vi "UHR-Fleezers Control (fpga) - 10.7.vi"() -> ()   [LabVIEW 2014]
doc: "UHR-Fleezers Instrument Control Code (fpga)"
uses:
  <vilib>/eio/EIONode/EIONode.xnode
  <vilib>/eio/EIOMethodNode/EIOMethodNode.xnode
  <vilib>/rvi/DataTransferAndStorage/Container/XNode/niFpgaContainer.xnode
  <vilib>/Platform/TimedLoop/XDataNode/XDataNode.xnode
  <vilib>/Platform/TimedLoop/XDataNode/nitl_modes.ctl
  <vilib>/Platform/TimedLoop/XDataNode/XDNodeRunTimeDep.lvlib
  <vilib>/Platform/TimedLoop/XDataNode/wakeup.ctl
  <vilib>/Platform/TimedLoop/XDataNode/timing_clust.ctl
  <vilib>/addons/control/pid/fpga.llb/XNode/niFpgaPID.xnode
  <vilib>/rvi/eio/common/nirviEmuTemplateMethod_errors.vi
  <vilib>/rvi/interface/RandomDataEmulation/nirviRandomDataFpgaReadWriteTemplate.vi
panel:
  in  "Connector0/AO6":i16
  in  "Tab Control":T1(tab)=enum."Force FB"
  in  "Trap Pos to FIFO":bool
  in  "AI1 Sets to FIFO":T2={"Set 1"=TRUE, "Set 2"=TRUE, "Set 3"=FALSE}
  in  "N of AI1 Int Acq Sets":i16=2 min=1 max=3 step=1
  out "AI Late Counter":u16
  in  "ai count":u32=400
  out "AI late?":bool
  in  "+ phase":bool
  in  "Phase count adjustment":i16
  out "Relative phase":i16
  in  "AI to FIFO":bool
  out "BD1 Frequency Out 1":u64
  out "BD1 Frequency Out 2":u64
  out "Trap Pos FIFO Timeout":u16
  out "Trap AI FIFO Timeout":u16
  in  "Trap FIFO Set Timeout":i32
  in  "Tab Control 2":T3(tab)
  out "Wiggling 2":bool
  in  "Abort wiggle 2":bool
  in  "Wiggle amp 2":u64
  in  "Wiggle freq 2 (Hz)":fxp<+/-,16,16>
  in  "Wiggle trap 2":bool
  out "Wiggling 1":bool
  in  "Abort wiggle 1":bool
  in  "Wiggle trap 1":bool
  in  "Wiggle amp 1":u64
  in  "Wiggle freq 1 (Hz)":fxp<+/-,16,16>
  in  "Swap F1 and F2":bool
  in  "Freq or Amp switch first":bool=TRUE
  in  "Cont. Scan":bool
  in  "Abort scan":bool
  in  "Cycles per step":u64
  in  "Scan BD":bool
  in  "Number of scans":u16
  in  "Scan steps":u64
  in  "Scan freq.  increment":i64
  out "Scanning":bool
  in  "Start scan":bool
  in  "OSK Bd 1":bool
  in  "Reset Bd 1":bool
  in  "RD":bool
  in  "PMODE":bool
  in  "OSK Bd 2":bool
  in  "Reset Bd 2":bool
  in  "Direct RF Box \nCommunication":bool
  in  "Data BD 2":u8 format="%08b"
  in  "Data BD 1":u8 format="%08b"
  in  "Address":u8 format="%02x"
  in  "Update Data":bool
  in  "FPGA Controls\n RF Box":bool
  in  "Number Interlace Cycles":u8=2 min=1 max=3
  in  "Interlace Off Parameters":u8=1 min=1 max=3
  in  "Interlace ON/OFF":bool
  out "DIO Relative phase":i16
  in  "Phase count adjustment (DIO)":i16
  in  "+ phase (DIO)":bool
  out "DIO Late Counter":u16
  out "DIO Late?":bool
  in  "DIO count 1 (ticks)":u32=400
  in  "DIO count 2 (ticks)":u32=400
  in  "DIO count 3 (ticks)":u32=400
  out "AI2 Y Sum Set 2":i16
  out "AI2 Y Sum Set 1":i16
  in  "FB Gains Set 1":T4={"proportional gain (Kc)"=10, "integral gain (Kc*Ts/Ti)"=5, "derivative gain (Kc*Td/Ts)"=0}
  in  "FB Setpoint Set 1":i16 min=0 step=1
  in  "FB Reset Set 1":bool
  in  "FB On/Off Set 1":bool
  in  "FB Reset Set 2":bool
  in  "FB On/Off Set 2":bool
  in  "FB Setpoint Set 2":i16 min=0 step=1
  in  "FB Gains Set 2":T4={"proportional gain (Kc)"=10, "integral gain (Kc*Ts/Ti)"=5, "derivative gain (Kc*Td/Ts)"=0}
  in  "FB output range 2":cluster{"output high":i16, "output low":i16}={"output high"=3000, "output low"=0}
  in  "FB output range 1":cluster{"output high":i16, "output low":i16}={"output high"=3000, "output low"=0}
  out "Scan I":u64
  in  "Amp switch delay":u16=5
  in  "Freq switch delay":u16
  in  "BD 2 Amplitude 1":u16
  in  "BD 1 Amplitude 1":u16
  in  "BD 2 Frequency 1":u64
  in  "BD 1 Frequency 1":u64
  in  "BD 2 Amplitude 2":u16
  in  "BD 1 Amplitude 2":u16
  in  "BD 2 Frequency 2":u64
  in  "BD 1 Frequency 2":u64
  in  "BD 2 Amplitude 3":u16
  in  "BD 1 Amplitude 3":u16
  in  "BD 2 Frequency 3":u64
  in  "BD 1 Frequency 3":u64
  in  "Negate Diff?":bool
  in  "Diff FB Measurement?":bool
  in  "FB Trig Integrate":u32=1
  out "TTrig?":bool
  in  "TTrig Negate Pos":bool=TRUE
  out "Trap Pos FB Int Signal":fxp<+/-,24,9> format="%.18g"
  out "Trap Pos FB Int-Norm Signal":fxp<+/-,16,1> format="%.16g"
  in  "FPGA TTrig Thresh":i64
  in  "FPGA Trap Trig":bool
  out "Trap Pos FB Action":i64
  in  "Trap Pos. FB Offset Factor":i64
  in  "Trap Pos. FB Mult Factor":i64=2
  in  "Trap Pos. FB Range":T5={"output high"=0.999969482421875, "output low"=-1.0}
  in  "Trap Pos. FB Gains":T6={"proportional gain (Kc)"=0.0, "integral gain (Kc*Ts/Ti)"=10.0, "derivative gain (Kc*Td/Ts)"=0.0} {"proportional gain (Kc)" format="%.11g"; "integral gain (Kc*Ts/Ti)" format="%.11g"; "derivative gain (Kc*Td/Ts)" format="%.11g"}
  in  "Trap Pos. FB Reset":bool
  in  "Trap Pos FB Monitor T1 or T2":bool
  in  "AI1 X Scale":u16
  in  "Trap Pos FB Int Count":u16=100
  in  "Trap Pos FB Negate Action":bool
  out "AI1 X Set 2":fxp<+/-,16,1>
  out "AI1 X Set 1":fxp<+/-,16,1>
  in  "Trap Pos. FB SP":fxp<+/-,16,1>
  in  "Force feedback":bool
  out "TTrig Sig":i64
  out "TTrig Fin Thresh":i64
  out "Numeric":i32
  out "AO2 2":i16
  out "AO1 2":i16
  in  "1D or 2D Scan?":bool
  in  "Abort scan (MCL)":bool
  in  "MCL Scan Axis":bool
  in  "Cont. Scan (MCL)":bool
  out "Scan I (MCL)":u64
  in  "Number of scans (MCL)":u16
  out "Scanning MCL":bool
  in  "Scan steps (MCL)":u64
  in  "Cycles per step (MCL)":u64
  in  "Scan freq.  increment (MCL)":i16
  in  "Start scan (MCL)":bool
  in  "AO2":i16
  in  "AO1":i16
  out "MCL Late Counter":u16
  out "MCL Late?":bool
  in  "MCL count":u32=800
  out "MCL Relative Phase":i16
  in  "Phase count adjustment (MCL)":i16
  in  "+ phase (MCL)":bool
  in  "APD Gate Operating Mode":u8 max=2 step=1
  in  "Invert APD Gate":bool
  in  "APD Gate OFF Count":u32=100
  in  "APD Gate ON Count":u32=300
  out "APD 1 Gate Late Counter":u16
  out "APD 1 Gate Late?":bool
  out "APD 1 Gate Relative Phase":i16
  in  "Phase count adjustment (APD 1 Gate)":i16
  in  "+ phase (APD 1 Gate)":bool
  out "APD 2 Counts 0":u32
  out "APD 2 Counts 1":u32
  out "APD 1 Counts 0":u32
  out "APD 1 Counts 1":u32
  out "APD 1 out state":bool
  in  "APD 2 AO scale factor":i16=1
  in  "APD 1 AO scale factor":i16=1
  in  "APD to FIFO":bool
  in  "APD Acq Rate Count":u32=20000000
  out "APD Acq Late Counter":u16
  out "APD Acq Late?":bool
  out "APD Acq Relative Phase":i16
  in  "Phase Count Adjustment (APD Acq)":i16
  in  "+ phase (APD Acq)":bool
  in  "Phase count adjustment (APD 2 Gate)":i16
  out "APD 2 Gate Late Counter":u16
  out "APD 2 Gate Late?":bool
  out "APD 2 Gate Relative Phase":i16
  in  "+ phase (APD 2 Gate)":bool
  out "APD 2 out state":bool
  out "APD 1 Int Gate":bool
  out "APD 2 Int Gate":bool
  in  "Green Filter Flipper":bool
  out "Green FB Signals":T7
  in  "Green FB Count":u32=1200
  out "Green Late Counter":u16
  out "Green FB Late?":bool
  out "Green FB Relative Phase":i16
  in  "Phase count adjustment (Green FB)":i16=10
  in  "+ phase (Green FB)":bool
  out "Green FB Sum":i16
  in  "Green int current ON count adj":u32=150
  in  "Current Out":u16=30000
  in  "Green FB On/Off":bool
  in  "Green FB Setpoint":i16=250 min=0 step=1
  in  "Green FB Gains":T4={"proportional gain (Kc)"=10, "integral gain (Kc*Ts/Ti)"=5, "derivative gain (Kc*Td/Ts)"=0}
  in  "Green FB Reset":bool
  in  "Operating Mode 2":u8=2 max=2 step=1
  in  "Invert GI 2":bool
  in  "Green interlace OFF count 2":u32=900
  in  "Green interlace ON count 2":u32=300
  out "GI Late Counter 2":u16
  out "GI Late? 2":bool
  out "GI Relative phase 2":i16
  in  "Phase count adjustment (GI) 2":i16=20
  in  "+ phase (GI) 2":bool
  in  "Green interlace OFF count":u32=100
  out "GI Relative phase":i16
  in  "Phase count adjustment (GI)":i16
  in  "+ phase (GI)":bool
  out "GI Late?":bool
  in  "Green interlace ON count":u32=300
  out "GI Late Counter":u16
  in  "Invert GI":bool
  in  "Operating Mode":u8 max=2 step=1
  in  "Chassis2/Mod4/AO1":u16
  # "Only one of these can be on\nat a time:"
  # "Raster Scan AOD"
  # "1 (X)"
  # "2 (Y)"
  # "IR Intensity Feedback (RF BD 1)"
  # "FB Triggering Excitation Laser"
  # "AO1 (Y)"
  # "2D"
  # "1D"
  # "AO2 (X)"
  # "APD AO for aligning"
  # "Detection Loop"
  # "Green fluorescent laser digital gate interlacing loop"
  # "0 Forced ON\n1 Forced OFF\n2 Interlacing"
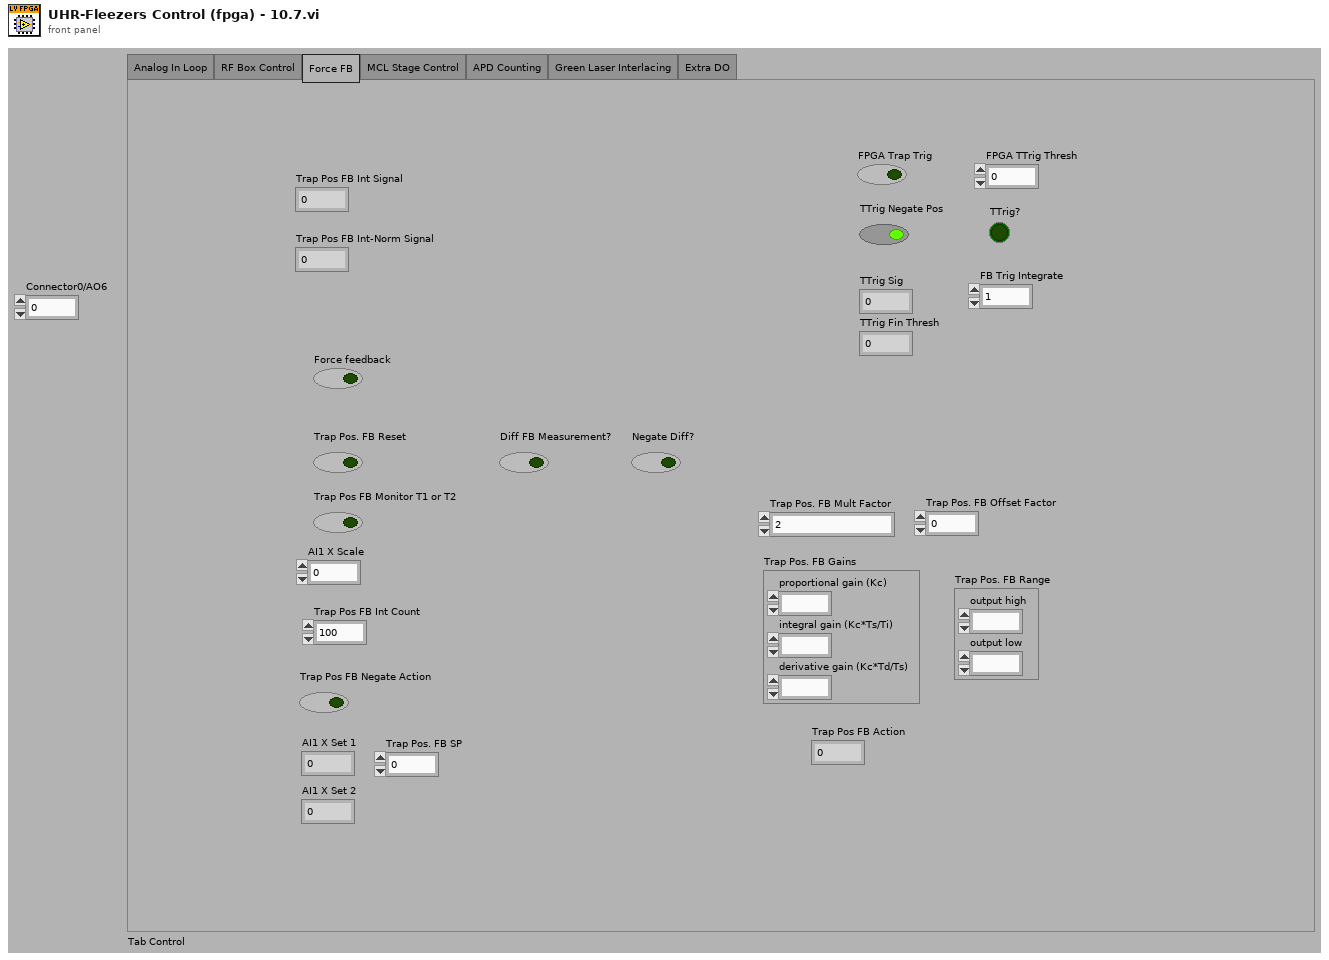
[diagram p1: front panel]
types:
  T1 = enum32{"Analog In Loop", "RF Box Control", "Force FB", "MCL Stage Control", "APD Counting", "Green Laser Interlacing", "Extra DO"}
  T2 = cluster{"Set 1":bool, "Set 2":bool, "Set 3":bool}
  T3 = enum32{"Controls", "Interlacing Frequency and Amplitude Values"}
  T4 = cluster{"proportional gain (Kc)":i16, "integral gain (Kc*Ts/Ti)":i16, "derivative gain (Kc*Td/Ts)":i16}
  T5 = cluster{"output high":fxp<+/-,16,1>, "output low":fxp<+/-,16,1>}
  T6 = cluster{"proportional gain (Kc)":fxp<+/-,16,8>, "integral gain (Kc*Ts/Ti)":fxp<+/-,16,8>, "derivative gain (Kc*Td/Ts)":fxp<+/-,16,8>}
  T7 = cluster{"Green FB Ch 0":i16, "Green FB Ch 1":i16, "Green FB Ch 2":i16}
  T8 = typedef "XDNodeRunTimeDep.lvlib/timing_clust.ctl" = cluster{"Expected End [f-1]":u64, "Actual End [f-1]":u64, "Finished Late? [f-1]":bool, "Expected End [i-1]":u64, "Actual End [i-1]":u64, "Finished Late? [i-1]":bool, "Expected Start [i]":u64, "Actual Start [i]":u64, "Expected Start [f]":u64, "Actual Start [f]":u64, "Source Name":string, "Structure Name":string, "Period":i64, "Deadline":i64, "Offset":i64, "Start":i64, "Priority":i32, "Timeout":i32, "Mode":T9, "Wakeup Reason":T10, "Error":errorcluster, "Source Type":string, "Secondary Source Type":string, "Global End Time":u64, "Global Start Time":u64, "Frame Duration":u64, "Iteration Duration":u64, "Assigned CPU":i32, "I/O Scan Engine Mode":u32}
  T9 = typedef "XDNodeRunTimeDep.lvlib/nitl_modes.ctl" = enum32{"No Change", "Process missed periods, maintain original phase", "Discard missed periods, maintain original phase", "Process missed periods, ignore original phase", "Discard missed periods, ignore original phase"}
  T10 = typedef "XDNodeRunTimeDep.lvlib/wakeup.ctl" = enum32{"Normal", "Aborted", "Asynchronous wakeup", "Timing source error", "Timed loop error", "Timeout"}
  T11 = cluster{"Chassis2/Mod1/AI0":void, "Chassis2/Mod1/AI1":void, "Chassis2/Mod1/AI2":void}
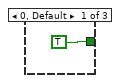
[diagram p2: hidden frame]
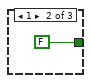
[diagram p3: hidden frame]
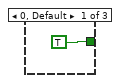
[diagram p5: hidden frame]
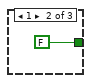
[diagram p6: hidden frame]
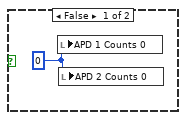
[diagram p7: hidden frame]
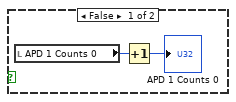
[diagram p10: hidden frame]
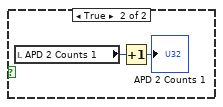
[diagram p12: hidden frame]
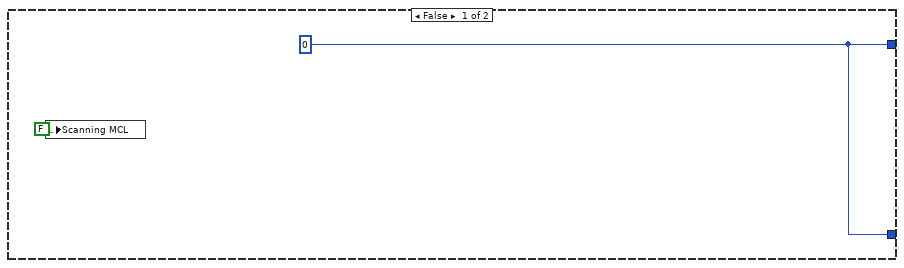
[diagram p13: hidden frame]
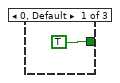
[diagram p14: hidden frame]
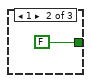
[diagram p15: hidden frame]
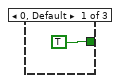
[diagram p16: hidden frame]
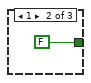
[diagram p17: hidden frame]
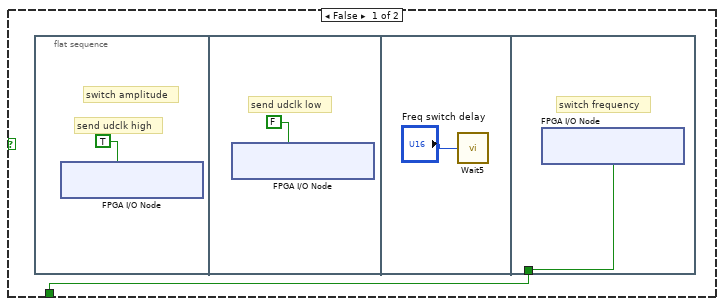
[diagram p20: hidden frame]
diagram:
  w3 = FALSE
  # "The APD Int Gate is here so the FPGA will do the integration only when the APD gate is \"ON\" (though we will leave the APD continuously ON now). This was added because the actual APD gating (via the hardware) was giving false signals. -KW"
  # "timing array current index"
  # "timing array"
  # "timing counter (phase adjusted here)"
  # "late counter"
  n1 = flat-sequence "FPGA initialization to do before running any of the loops" {
    tunnel: [u32 0 ("DIO count 3 (ticks)")] -> w2
    tunnel: [w10] -> _
    frame #0 {
      # "Start up expansion chassis early\nto avoid delays later"
      # "This pin controls udclk on the RF boards.\nWhen initially configuring the boards, this pin needs to be\nconfigured as a high impedance input.  Later it will be switched\nto an output."
      # "Initial setting of DIO data and \naddress to low (before reset).  \nThis needs to happen before the other\ncontrol method loops execute."
      n2 = xnode "FPGA I/O Node"("Chassis2/Mod4/AO0"=u16 0) -> ("Chassis2/Mod1/AI0"=w10)  [unwired: 2 in, 2 out]
      n3 = xnode "FPGA I/O Method Node"("Enable"=FALSE) -> ()  [unwired: 1 in, 1 out]
      n4 = xnode "FPGA I/O Node"("Connector1/DIO0"=FALSE, "Connector1/DIO1"=FALSE, "Connector1/DIO2"=FALSE, "Connector1/DIO3"=FALSE, "Connector1/DIO4"=FALSE, "Connector1/DIO5"=FALSE, "Connector1/DIO6"=FALSE, "Connector1/DIO7"=FALSE, "Connector1/DIO8"=FALSE, "Connector1/DIO9"=FALSE, "Connector1/DIO10"=FALSE, "Connector1/DIO11"=FALSE, "Connector1/DIO12"=FALSE, "Connector1/DIO13"=FALSE, "Connector1/DIO15"=FALSE, "Connector1/DIO20"=FALSE, "Connector1/DIO21"=FALSE, "Connector1/DIO22"=FALSE, "Connector1/DIO23"=FALSE, "Connector1/DIO24"=FALSE, "Connector1/DIO25"=FALSE, "Connector1/DIO26"=FALSE, "Connector1/DIO27"=FALSE, "Connector1/DIO14"=FALSE) -> ()  [unwired: 24 in, 24 out]
    }
  }
  n5 = local read "AO1"() -> (w7:i16)
  n6 = local read "AO2"() -> (w6:i16)
  n7 = node-c288() -> (w5:T8)  [unwired: 1 in]
  n8 = while "APD 1 Counter" {
    tunnel: w2 -> [_]
    stop <- FALSE stop-if-true
    n9 = flat-sequence {
      frame #0 {
        n10 = xnode "FPGA I/O Method Node"("FPGA I/O In"=refnum<k21> "Connector0/DIO0" ("APD 1 DO"), "Timeout"=-1) -> ()  [unwired: 2 out]
      }
      frame #1 {
        n11 = local read "APD 1 Int Gate"() -> (w41:bool)
        n12 = case shown="True" w41 {
          frame False {
          }
          frame True {
            n13 = local read "APD 1 out state"() -> (w42:bool)
            n14 = case shown="True" w42 {
              frame False {
                n15 = local read "APD 1 Counts 0"() -> (w44:u32)
                n16 = Increment(x=w44) -> (x+1=→"APD 1 Counts 0":u32)
              }
              frame True {
                n17 = local read "APD 1 Counts 1"() -> (w46:u32)
                n18 = Increment(x=w46) -> (x+1=→"APD 1 Counts 1":u32)
              }
            }
          }
        }
      }
    }
  }
  n19 = while "APD 2 Counter" {
    tunnel: w2 -> [_]
    stop <- FALSE stop-if-true
    n20 = flat-sequence {
      frame #0 {
        n21 = xnode "FPGA I/O Method Node"("FPGA I/O In"=refnum<k21> "Connector0/DIO1" ("APD 2 DO"), "Timeout"=-1) -> ()  [unwired: 2 out]
      }
      frame #1 {
        n22 = local read "APD 2 Int Gate"() -> (w50:bool)
        n23 = case shown="True" w50 {
          frame False {
          }
          frame True {
            n24 = local read "APD 2 out state"() -> (w51:bool)
            n25 = case shown="False" w51 {
              frame False {
                n26 = local read "APD 2 Counts 0"() -> (w53:u32)
                n27 = Increment(x=w53) -> (x+1=→"APD 2 Counts 0":u32)
              }
              frame True {
                n28 = local read "APD 2 Counts 1"() -> (w55:u32)
                n29 = Increment(x=w55) -> (x+1=→"APD 2 Counts 1":u32)
              }
            }
          }
        }
      }
    }
  }
  n30 = while "APD 2 Gating" {
    shift-right: [w59] -> _
    shift-left: w2 -> [w64]
    shift-right: [w58] -> _
    shift-left: w3 -> [w56]
    stop <- FALSE stop-if-true
    n31 = flat-sequence {
      tunnel: w64 -> [w67]
      tunnel: [w68] -> w62
      tunnel: [w67] -> w60
      tunnel: [w66] -> w57
      tunnel: w56 -> [w66]
      tunnel: [w71] -> w63
      tunnel: w62 -> [w71]
      tunnel: [w70] -> w61
      tunnel: w60 -> [w70]
      tunnel: w57 -> [w69]
      tunnel: [w89] -> w59
      tunnel: w63 -> [w100]
      tunnel: w61 -> [w98]
      tunnel: [w93] -> w58
      frame #0 {
        n32 = call "Loop Timer8"("Count(Ticks)"=w67) -> ("Tick Count(Ticks)"=w68:u32)
      }
      frame #1 {
        # "(need 4 channels/APD)"
        n33 = xnode "FPGA I/O Node"("Connector0/DIO8"=w69, "Connector0/DIO9"=w69, "Connector0/DIO10"=w69, "Connector0/DIO11"=w69) -> ()  [unwired: 4 in, 4 out]
        "APD 2 Int Gate" <- w69
      }
      frame #2 {
        n34 = local read "APD Gate ON Count"() -> (w82:u32)
        n35 = local read "APD Gate OFF Count"() -> (w81:u32)
        n36 = feedback #1(TRUE) -> (w95:bool)
        n37 = feedback-in #2(w100) -> ()
        n38 = feedback #2(w100) -> (w83:u32)
        n39 = Not(x=w95) -> (.not. x?=w92:bool)
        n40 = feedback-in #1(w92) -> ()
        n41 = Subtract(x=w100, y=w83) -> (x-y=w99:u32)
        n42 = Select(t=w82, s=w92, f=w81) -> (s? t:f=w97:u32)
        n43 = Subtract(x=w99, y=w98) -> (x-y=w74:u32)
        n44 = Subtract(x=w97, y=w74) -> (x-y=w88:u32)
        n45 = Number To Boolean Array(number=w74) -> (Boolean array=w73:bool[])
        n46 = Or Array Elements(Boolean array=w73) -> (logical OR=w72:bool)
        "APD 2 Gate Late?" <- w72
        n47 = Boolean To (0,1)(Boolean="+ phase (APD 2 Gate)") -> (0, 1=w86:i16)
        n48 = Multiply(x=w86, y="Phase count adjustment (APD 2 Gate)") -> (x*y=w84:i16)
        n49 = Boolean To (0,1)(Boolean=w72) -> (0, 1=w79:i16)
        n50 = Add(x=w88, y=w84) -> (x+y=w89:u32)
        n51 = To Unsigned Word Integer(number=w79) -> (unsigned 16bit integer=w76:u16)
        n52 = feedback #3(i16 0) -> (w91:i16)
        n53 = Subtract(x=w91, y=w84) -> (x-y=w90:i16)
        "APD 2 Gate Relative Phase" <- w90
        n54 = feedback-in #3(w90) -> ()
        n55 = feedback #4(u16 0) -> (w77:u16)
        n56 = Add(x=w76, y=w77) -> (x+y=w75:u16)
        "APD 2 Gate Late Counter" <- w75
        n57 = feedback-in #4(w75) -> ()
        n58 = local read "APD Gate Operating Mode"() -> (w80:u8)
        n59 = case shown="2" w80 {
          tunnel: [TRUE FALSE w106] -> w93
          tunnel: w95 -> [_ _ w104]
          frame 0, Default {
          }
          frame 1 {
          }
          frame 2 {
            n60 = local read "Invert APD Gate"() -> (w103:bool)
            n61 = Not(x=w104) -> (.not. x?=w105:bool)
            n62 = Select(t=w105, s=w103, f=w104) -> (s? t:f=w106:bool)
          }
        }
      }
    }
  }
  n63 = while "APD 1 Gating" {
    shift-right: [w110] -> _
    shift-left: w2 -> [w115]
    shift-right: [w109] -> _
    shift-left: w3 -> [w107]
    stop <- FALSE stop-if-true
    n64 = flat-sequence {
      tunnel: w115 -> [w118]
      tunnel: [w119] -> w113
      tunnel: [w118] -> w111
      tunnel: [w117] -> w108
      tunnel: w107 -> [w117]
      tunnel: [w122] -> w114
      tunnel: w113 -> [w122]
      tunnel: [w121] -> w112
      tunnel: w111 -> [w121]
      tunnel: w108 -> [w120]
      tunnel: [w136] -> w110
      tunnel: w114 -> [w151]
      tunnel: w112 -> [w148]
      tunnel: [w140] -> w109
      frame #0 {
        n65 = call "Loop Timer7"("Count(Ticks)"=w118) -> ("Tick Count(Ticks)"=w119:u32)
      }
      frame #1 {
        # "(need 4 channels/APD)"
        n66 = xnode "FPGA I/O Node"("Connector0/DIO4"=w120, "Connector0/DIO5"=w120, "Connector0/DIO6"=w120, "Connector0/DIO7"=w120) -> ()  [unwired: 4 in, 4 out]
        "APD 1 Int Gate" <- w120
      }
      frame #2 {
        n67 = feedback #5(TRUE) -> (w143:bool)
        n68 = feedback-in #6(w151) -> ()
        n69 = feedback #6(w151) -> (w150:u32)
        n70 = Not(x=w143) -> (.not. x?=w139:bool)
        n71 = feedback-in #5(w139) -> ()
        n72 = Subtract(x=w151, y=w150) -> (x-y=w149:u32)
        n73 = Select(t="APD Gate ON Count", s=w139, f="APD Gate OFF Count") -> (s? t:f=w145:u32)
        n74 = Subtract(x=w149, y=w148) -> (x-y=w124:u32)
        n75 = Subtract(x=w145, y=w124) -> (x-y=w135:u32)
        n76 = Number To Boolean Array(number=w124) -> (Boolean array=w125:bool[])
        n77 = Or Array Elements(Boolean array=w125) -> (logical OR=w123:bool)
        "APD 1 Gate Late?" <- w123
        n78 = Boolean To (0,1)(Boolean="+ phase (APD 1 Gate)") -> (0, 1=w133:i16)
        n79 = Boolean To (0,1)(Boolean=w123) -> (0, 1=w130:i16)
        n80 = Multiply(x=w133, y="Phase count adjustment (APD 1 Gate)") -> (x*y=w131:i16)
        n81 = To Unsigned Word Integer(number=w130) -> (unsigned 16bit integer=w127:u16)
        n82 = Add(x=w135, y=w131) -> (x+y=w136:u32)
        n83 = feedback #7(i16 0) -> (w138:i16)
        n84 = Subtract(x=w138, y=w131) -> (x-y=w137:i16)
        "APD 1 Gate Relative Phase" <- w137
        n85 = feedback-in #7(w137) -> ()
        n86 = feedback #8(u16 0) -> (w128:u16)
        n87 = Add(x=w127, y=w128) -> (x+y=w126:u16)
        "APD 1 Gate Late Counter" <- w126
        n88 = feedback-in #8(w126) -> ()
        n89 = case shown="2" "APD Gate Operating Mode" {
          tunnel: [TRUE FALSE w157] -> w140
          tunnel: w143 -> [_ _ w154]
          frame 0, Default {
          }
          frame 1 {
          }
          frame 2 {
            n90 = Not(x=w154) -> (.not. x?=w156:bool)
            n91 = Select(t=w156, s="Invert APD Gate", f=w154) -> (s? t:f=w157:bool)
          }
        }
      }
    }
  }
  n92 = timed-loop "RF box board DIO control: control bits" {
    timing: w5 -> [_]
    timing-out: [_] -> w4
    tunnel: [w158] -> _
    tunnel: w2 -> [w158]
    stop <- FALSE stop-if-true
    n93 = xnode "FPGA I/O Node"("Connector1/DIO16"="RD", "Connector1/DIO17"="PMODE", "Connector1/DIO18"="OSK Bd 1", "Connector1/DIO19"="Reset Bd 1", "Connector1/DIO28"="OSK Bd 2", "Connector1/DIO29"="Reset Bd 2") -> ()  [unwired: 6 in, 6 out]
  }
  n94 = while "Green fluorescent laser interlacing (DO to IA 532 nm AOM ME amp)." {
    shift-right: [w171] -> _
    shift-left: w2 -> [w176]
    shift-right: [w170] -> _
    shift-left: FALSE -> [w168]
    stop <- FALSE stop-if-true
    n95 = flat-sequence {
      tunnel: w176 -> [w179]
      tunnel: [w180] -> w174
      tunnel: [w179] -> w172
      tunnel: [w178] -> w169
      tunnel: w168 -> [w178]
      tunnel: [w183] -> w175
      tunnel: w174 -> [w183]
      tunnel: [w182] -> w173
      tunnel: w172 -> [w182]
      tunnel: w169 -> [w181]
      tunnel: [w192] -> w171
      tunnel: w175 -> [w212]
      tunnel: w173 -> [w209]
      tunnel: [w201] -> w170
      frame #0 {
        n96 = call "Loop Timer4"("Count(Ticks)"=w179) -> ("Tick Count(Ticks)"=w180:u32)
      }
      frame #1 {
        n97 = xnode "FPGA I/O Node"("Connector1/DIO37"=w181, "Connector1/DIO38"=w181, "Connector1/DIO39"=w181) -> ()  [unwired: 3 in, 3 out]
      }
      frame #2 {
        n98 = feedback-in #9(w212) -> ()
        n99 = feedback #9(w212) -> (w211:u32)
        n100 = Subtract(x=w212, y=w211) -> (x-y=w210:u32)
        n101 = Subtract(x=w210, y=w209) -> (x-y=w185:u32)
        n102 = Number To Boolean Array(number=w185) -> (Boolean array=w186:bool[])
        n103 = Or Array Elements(Boolean array=w186) -> (logical OR=w184:bool)
        "GI Late?" <- w184
        n104 = Boolean To (0,1)(Boolean="+ phase (GI)") -> (0, 1=w197:i16)
        n105 = Multiply(x=w197, y="Phase count adjustment (GI)") -> (x*y=w194:i16)
        n106 = Boolean To (0,1)(Boolean=w184) -> (0, 1=w191:i16)
        n107 = To Unsigned Word Integer(number=w191) -> (unsigned 16bit integer=w188:u16)
        n108 = feedback #10(i16 0) -> (w195:i16)
        n109 = feedback #11(u16 0) -> (w189:u16)
        n110 = Add(x=w188, y=w189) -> (x+y=w187:u16)
        "GI Late Counter" <- w187
        n111 = feedback-in #11(w187) -> ()
        n112 = Subtract(x=w195, y=w194) -> (x-y=w193:i16)
        "GI Relative phase" <- w193
        n113 = feedback-in #10(w193) -> ()
        n114 = feedback #12(TRUE) -> (w204:bool)
        n115 = case shown="2" "Operating Mode" {
          tunnel: [TRUE FALSE w218] -> w201
          tunnel: w204 -> [_ _ w215]
          frame 0, Default {
          }
          frame 1 {
          }
          frame 2 {
            n116 = Not(x=w215) -> (.not. x?=w217:bool)
            n117 = Select(t=w217, s="Invert GI", f=w215) -> (s? t:f=w218:bool)
          }
        }
        n118 = Not(x=w204) -> (.not. x?=w200:bool)
        n119 = Select(t="Green interlace ON count", s=w200, f="Green interlace OFF count") -> (s? t:f=w206:u32)
        n120 = Subtract(x=w206, y=w185) -> (x-y=w198:u32)
        n121 = Add(x=w198, y=w194) -> (x+y=w192:u32)
        n122 = feedback-in #12(w200) -> ()
      }
    }
  }
  n123 = while "Green fluorescent laser interlacing (Current to IA 532 nm AOM ME amp)." {
    shift-right: [w224] -> _
    shift-left: w2 -> [w227]
    shift-right: [w221] -> _
    shift-left: u16 0 -> [w219]
    stop <- FALSE stop-if-true
    n124 = flat-sequence {
      tunnel: w227 -> [w230]
      tunnel: [w231] -> w226
      tunnel: [w230] -> w225
      tunnel: [w229] -> w220
      tunnel: w219 -> [w229]
      tunnel: [w234] -> w223
      tunnel: w226 -> [w234]
      tunnel: [w233] -> w222
      tunnel: w225 -> [w233]
      tunnel: w220 -> [w232]
      tunnel: [w243] -> w224
      tunnel: [w260] -> w221
      tunnel: w223 -> [w273]
      tunnel: w222 -> [w270]
      frame #0 {
        n125 = call "Loop Timer10"("Count(Ticks)"=w230) -> ("Tick Count(Ticks)"=w231:u32)
      }
      frame #1 {
        n126 = xnode "FPGA I/O Node"("Chassis2/Mod4/AO0"=w232) -> ()  [unwired: 1 in, 1 out]
      }
      frame #2 {
        n127 = Subtract(x="Green interlace OFF count 2", y="Green int current ON count adj") -> (x-y=w252:u32)
        n128 = feedback-in #13(w273) -> ()
        n129 = feedback #13(w273) -> (w272:u32)
        n130 = Add(x="Green int current ON count adj", y="Green interlace ON count 2") -> (x+y=w253:u32)
        n131 = Subtract(x=w273, y=w272) -> (x-y=w271:u32)
        n132 = Subtract(x=w271, y=w270) -> (x-y=w236:u32)
        n133 = Number To Boolean Array(number=w236) -> (Boolean array=w237:bool[])
        n134 = Boolean To (0,1)(Boolean="+ phase (GI) 2") -> (0, 1=w249:i16)
        n135 = Or Array Elements(Boolean array=w237) -> (logical OR=w235:bool)
        "GI Late? 2" <- w235
        n136 = Boolean To (0,1)(Boolean=w235) -> (0, 1=w242:i16)
        n137 = Multiply(x=w249, y="Phase count adjustment (GI) 2") -> (x*y=w245:i16)
        n138 = To Unsigned Word Integer(number=w242) -> (unsigned 16bit integer=w238:u16)
        n139 = feedback #14(u16 0) -> (w240:u16)
        n140 = Add(x=w238, y=w240) -> (x+y=w239:u16)
        "GI Late Counter 2" <- w239
        n141 = feedback-in #14(w239) -> ()
        n142 = feedback #15(i16 0) -> (w246:i16)
        n143 = Subtract(x=w246, y=w245) -> (x-y=w244:i16)
        "GI Relative phase 2" <- w244
        n144 = feedback-in #15(w244) -> ()
        n145 = feedback #16(TRUE) -> (w265:bool)
        n146 = case shown="2" "Operating Mode 2" {
          tunnel: [TRUE FALSE w290] -> w254
          tunnel: w265 -> [_ _ w287]
          frame 0, Default {
          }
          frame 1 {
          }
          frame 2 {
            n147 = Not(x=w287) -> (.not. x?=w289:bool)
            n148 = Select(t=w289, s="Invert GI 2", f=w287) -> (s? t:f=w290:bool)
          }
        }
        n149 = And(x=w254, y="Green FB On/Off") -> (x .and. y?=w255:bool)
        n150 = case shown="True" w255 {
          tunnel: "Current Out" -> [w274 _]
          tunnel: [w274 w279] -> w259
          frame False {
          }
          frame True {
            n151 = local read "Green FB Sum"() -> (w275:i16)
            n152 = call "Slower PID.vi"("process variable"=w275, "reset?"="Green FB Reset", "setpoint"="Green FB Setpoint", "PID gains (x 2^8)"="Green FB Gains", "output range"=cluster{"output high":i16, "output low":i16} {"output high"=32767, "output low"=-32768} ("Green FB output range")) -> ("output"=w283:i16)  [unwired: 10 out]
            n153 = To Long Integer(number=w283) -> (32bit integer=w276:i32)
            n154 = Add(x=w276, y=32768) -> (x+y=w278:i32)
            n155 = To Unsigned Word Integer(number=w278) -> (unsigned 16bit integer=w279:u16)
          }
        }
        n156 = Not(x=w265) -> (.not. x?=w262:bool)
        n157 = Select(t=w253, s=w262, f=w252) -> (s? t:f=w267:u32)
        n158 = Subtract(x=w267, y=w236) -> (x-y=w247:u32)
        n159 = Add(x=w247, y=w245) -> (x+y=w243:u32)
        n160 = feedback-in #16(w262) -> ()
        n161 = Boolean To (0,1)(Boolean=w254) -> (0, 1=w261:i16)
        n162 = To Unsigned Word Integer(number=w261) -> (unsigned 16bit integer=w258:u16)
        n163 = Multiply(x=w258, y=w259) -> (x*y=w260:u16)
      }
    }
  }
  n164 = while "Green excitation laser feedback measurement" {
    shift-right: [w291] -> _
    shift-left: w2 -> [w296]
    stop <- FALSE stop-if-true
    n165 = flat-sequence {
      tunnel: w296 -> [w298]
      tunnel: [w299] -> w294
      tunnel: [w298] -> w292
      tunnel: [w306] -> w295
      tunnel: w294 -> [w306]
      tunnel: [w305] -> w293
      tunnel: w292 -> [w305]
      tunnel: [w318] -> w291
      tunnel: w295 -> [w329]
      tunnel: w293 -> [w326]
      frame #0 {
        n166 = call "Loop Timer9"("Count(Ticks)"=w298) -> ("Tick Count(Ticks)"=w299:u32)
      }
      frame #1 {
        n167 = xnode "FPGA I/O Node"("Connector1/DIO35"=TRUE) -> ("Chassis2/Mod1/AI0"=w304, "Chassis2/Mod1/AI1"=w303, "Chassis2/Mod1/AI2"=w300)  [unwired: 4 in, 4 out]
        "Green FB Sum" <- w300
        n168 = Bundle("Chassis2/Mod1/AI0"=w304, "Chassis2/Mod1/AI1"=w303, "Chassis2/Mod1/AI2"=w300) -> (→"Green FB Signals":T11)  [unwired: 1 out]
      }
      frame #2 {
        n169 = feedback-in #17(w329) -> ()
        n170 = feedback #17(w329) -> (w328:u32)
        n171 = Subtract(x=w329, y=w328) -> (x-y=w327:u32)
        n172 = xnode "FPGA I/O Node"("Connector1/DIO35"=FALSE) -> ()  [unwired: 1 in, 1 out]
        n173 = Subtract(x=w327, y=w326) -> (x-y=w308:u32)
        n174 = Subtract(x="Green FB Count", y=w308) -> (x-y=w322:u32)
        n175 = Number To Boolean Array(number=w308) -> (Boolean array=w309:bool[])
        n176 = Or Array Elements(Boolean array=w309) -> (logical OR=w307:bool)
        "Green FB Late?" <- w307
        n177 = Boolean To (0,1)(Boolean="+ phase (Green FB)") -> (0, 1=w320:i16)
        n178 = Boolean To (0,1)(Boolean=w307) -> (0, 1=w314:i16)
        n179 = Multiply(x=w320, y="Phase count adjustment (Green FB)") -> (x*y=w315:i16)
        n180 = Add(x=w322, y=w315) -> (x+y=w318:u32)
        n181 = To Unsigned Word Integer(number=w314) -> (unsigned 16bit integer=w311:u16)
        n182 = feedback #18(i16 0) -> (w317:i16)
        n183 = Subtract(x=w317, y=w315) -> (x-y=w316:i16)
        "Green FB Relative Phase" <- w316
        n184 = feedback-in #18(w316) -> ()
        n185 = feedback #19(u16 0) -> (w312:u16)
        n186 = Add(x=w311, y=w312) -> (x+y=w310:u16)
        "Green Late Counter" <- w310
        n187 = feedback-in #19(w310) -> ()
      }
    }
  }
  n188 = while "Control Additional IO (Green laser flip mount)" {
    stop <- FALSE stop-if-true
    n189 = xnode "FPGA I/O Node"("Connector0/DIO3"="Green Filter Flipper", "Chassis2/Mod4/AO1"="Chassis2/Mod4/AO1", "Connector0/AO6"="Connector0/AO6") -> ()  [unwired: 3 in, 3 out]
    n190 = call "Loop Timer2"("Count(Ticks)"=u32 40000 ("Extra DO Counts")) -> ()  [unwired: 1 out]
  }
  n191 = while "DAQ AI set 1" {
    shift-right: [w335] -> _
    shift-left: w2 -> [w340]
    stop <- FALSE stop-if-true
    n192 = flat-sequence {
      tunnel: w340 -> [w350]
      tunnel: [w351] -> w338
      tunnel: [w350] -> w337
      tunnel: [w361] -> w348
      tunnel: [w360] -> w347
      tunnel: [w359] -> w346
      tunnel: [w358] -> w345
      tunnel: [w357] -> w344
      tunnel: [w356] -> w343
      tunnel: [w355] -> w342
      tunnel: [w354] -> w341
      tunnel: [w353] -> w339
      tunnel: w338 -> [w353]
      tunnel: w337 -> [w352]
      tunnel: [w352] -> w336
      tunnel: [w390] -> w335
      tunnel: w348 -> [w418]
      tunnel: w347 -> [w382]
      tunnel: w346 -> [w383]
      tunnel: w345 -> [w417]
      tunnel: w344 -> [w406]
      tunnel: w343 -> [w405]
      tunnel: w342 -> [w404]
      tunnel: w341 -> [w403]
      tunnel: w339 -> [w400]
      tunnel: w336 -> [w397]
      frame #0 {
        n193 = call "Loop Timer3"("Count(Ticks)"=w350) -> ("Tick Count(Ticks)"=w351:u32)
      }
      frame #1 {
        n194 = xnode "FPGA I/O Node"("Connector1/DIO31"=TRUE ("Connector1/DIO33")) -> ("Connector0/AI0"=w361, "Connector0/AI1"=w360, "Connector0/AI2"=w359, "Connector0/AI3"=w358, "Connector0/AI4"=w357, "Connector0/AI5"=w356, "Connector0/AI6"=w355, "Connector0/AI7"=w354)  [unwired: 9 in, 9 out]
      }
      frame #2 {
        w386 = FALSE ("AI to FIFO")
        # "Adjust phase after data acquired if button pressed"
        n195 = feedback #20(i16 1) -> (w410:i16)
        n196 = Increment(x=w410) -> (x+1=w416:i16)
        n197 = Scale By Power Of 2(n="AI1 X Scale", x=w382) -> (x*2^n=w380:dbl)
        n198 = Greater?(x=w416, y="N of AI1 Int Acq Sets") -> (0:w413:bool)
        n199 = Select(t=i16 1, s=w413, f=w416) -> (s? t:f=w415:i16)
        n200 = feedback-in #20(w415) -> ()
        n201 = Divide(x=w380, y=w383) -> (x/y=w379:fxp<+/-,16,1>)
        n202 = feedback #21(w386) -> (w384:bool)
        n203 = feedback #22(w386) -> (w402:bool)
        n204 = case shown="1, Default" w410 {
          tunnel: w383 -> [w440 w448 _]
          tunnel: "AI1 Sets to FIFO" -> [w444 w452 w458]
          tunnel: [w443 w451 w457] -> w407
          tunnel: ["AI to FIFO" w450 w456] -> w401
          tunnel: w402 -> [_ w450 w456]
          tunnel: ["Trap Pos to FIFO" w449 w455] -> w385
          tunnel: w384 -> [_ w449 w455]
          tunnel: w379 -> [w439 w447 _]
          tunnel: [w438 w445 FALSE] -> w366
          tunnel: [w437 w446 u64 0 ("BD1 Frequency Out 2")] -> w365
          frame 1, Default {
            n205 = Unbundle By Name(w444) -> ("Set 1"=w443:bool)
            n206 = local read "BD1 Frequency Out 1"() -> (w437:u64)
            n207 = Compound Arithmetic op=AND("Trap Pos to FIFO", w443, "AI to FIFO") -> (w438:bool)
            "AI2 Y Sum Set 1" <- w440
            "AI1 X Set 1" <- w439
          }
          frame 2 {
            n208 = Unbundle By Name(w452) -> ("Set 2"=w451:bool)
            n209 = local read "BD1 Frequency Out 2"() -> (w446:u64)
            n210 = Compound Arithmetic op=AND(w449, w451, w450) -> (w445:bool)
            "AI2 Y Sum Set 2" <- w448
            "AI1 X Set 2" <- w447
          }
          frame 3 {
            n211 = Unbundle By Name(w458) -> ("Set 3"=w457:bool)
          }
        }
        n212 = And(x=w407, y=w401) -> (x .and. y?=w409:bool)
        n213 = case shown="True" w409 {
          tunnel: w418 -> [_ w472]
          tunnel: w382 -> [_ w471]
          tunnel: w383 -> [_ w470]
          tunnel: w417 -> [_ w469]
          tunnel: w406 -> [_ w468]
          tunnel: w405 -> [_ w467]
          tunnel: w404 -> [_ w466]
          tunnel: w403 -> [_ w465]
          tunnel: 0 ("DMA buffer timeout") -> [_ w474]
          frame False {
          }
          frame True {
            n214 = Build Array(w472, w471, w470, w469, w468, w467, w466, w465) -> (w473:void[])
            n215 = for {
              tunnel: w473 -> [w476] mode=indexing
              tunnel: w474 -> [w477]
              tunnel: [w475] -> w463 mode=indexing
              n216 = xnode ("FIFO Write")("Element"=w476, "Timeout"=w477) -> ("Timed Out?"=w475:bool)  [unwired: 1 in, 1 out]
            }
            n217 = Or Array Elements(Boolean array=w463) -> (logical OR=w460:bool)
            n218 = Boolean To (0,1)(Boolean=w460) -> (0, 1=w462:i16)
            n219 = feedback #23(u16 0) -> (w461:u16)
            n220 = Add(x=w462, y=w461) -> (x+y=w459:u16)
            "Trap AI FIFO Timeout" <- w459
            n221 = feedback-in #23(w459) -> ()
          }
        }
        n222 = feedback-in #21(w385) -> ()
        n223 = feedback-in #22(w401) -> ()
        n224 = case shown="True" w366 {
          tunnel: w365 -> [_ w424]
          tunnel: [u8 0 w421] -> w364
          frame False {
          }
          frame True {
            n225 = Split Number(x=w424) -> (hi(x)=w425:u32, lo(x)=w426:u32)
            n226 = Split Number(x=w425) -> (lo(x)=w427:u16)  [unwired: 1 out]
            n227 = Split Number(x=w426) -> (hi(x)=w428:u16, lo(x)=w429:u16)
            n228 = Build Array "BD 1 nu Stack"(w427, w428, w429) -> (w423:u16[])
            n229 = for {
              tunnel: w423 -> [w436] mode=indexing
              shift-right: [w432] -> w421
              shift-left: u8 0 -> [w433]
              n230 = xnode ("FIFO Method Node")("Element"=w436, "Timeout"="Trap FIFO Set Timeout") -> ("Timed Out?"=w435:bool)  [unwired: 1 in, 1 out]
              n231 = Boolean To (0,1)(Boolean=w435) -> (0, 1=w434:i16)
              n232 = To Unsigned Byte Integer(number=w434) -> (unsigned 8bit integer=w431:u8)
              n233 = Add(x=w431, y=w433) -> (x+y=w432:u8)
            }
          }
        }
        n234 = To Unsigned Word Integer(number=w364) -> (unsigned 16bit integer=w363:u16)
        n235 = feedback #24(u16 0) -> (w377:u16)
        n236 = Add(x=w363, y=w377) -> (x+y=w376:u16)
        "Trap Pos FIFO Timeout" <- w376
        n237 = feedback-in #24(w376) -> ()
        n238 = feedback-in #25(w400) -> ()
        n239 = feedback #25(w400) -> (w399:u32)
        n240 = Subtract(x=w400, y=w399) -> (x-y=w398:u32)
        n241 = xnode "I/O Node"("Connector1/DIO31"=FALSE ("Connector1/DIO34")) -> ()  [unwired: 1 in, 1 out]
        n242 = Subtract(x=w398, y=w397) -> (x-y=w368:u32)
        n243 = Boolean To (0,1)(Boolean="+ phase") -> (0, 1=w393:i16)
        n244 = Multiply(x=w393, y="Phase count adjustment") -> (x*y=w387:i16)
        n245 = Subtract(x="ai count", y=w368) -> (x-y=w391:u32)
        n246 = Number To Boolean Array(number=w368) -> (Boolean array=w369:bool[])
        n247 = feedback #26(i16 0) -> (w389:i16)
        n248 = Add(x=w391, y=w387) -> (x+y=w390:u32)
        n249 = Subtract(x=w389, y=w387) -> (x-y=w388:i16)
        "Relative phase" <- w388
        n250 = feedback-in #26(w388) -> ()
        n251 = Or Array Elements(Boolean array=w369) -> (logical OR=w367:bool)
        "AI late?" <- w367
        n252 = Boolean To (0,1)(Boolean=w367) -> (0, 1=w374:i16)
        n253 = To Unsigned Word Integer(number=w374) -> (unsigned 16bit integer=w371:u16)
        n254 = feedback #27(u16 0) -> (w372:u16)
        n255 = Add(x=w371, y=w372) -> (x+y=w370:u16)
        "AI Late Counter" <- w370
        n256 = feedback-in #27(w370) -> ()
      }
    }
  }
  n257 = while "MCL stage control" {
    shift-right: [w493] -> _
    shift-left: w2 -> [w496]
    shift-right: [w486] -> _
    shift-left: w7 -> [w483]
    shift-right: [w485] -> _
    shift-left: w6 -> [w481]
    i -> [w480]
    stop <- FALSE stop-if-true
    n258 = flat-sequence {
      tunnel: w496 -> [w500]
      tunnel: [w501] -> w492
      tunnel: [w500] -> w490
      tunnel: [w499] -> w484
      tunnel: w483 -> [w499]
      tunnel: [w498] -> w482
      tunnel: w481 -> [w498]
      tunnel: w492 -> [w505]
      tunnel: [w505] -> w491
      tunnel: w490 -> [w504]
      tunnel: [w504] -> w489
      tunnel: w484 -> [w503]
      tunnel: w482 -> [w502]
      tunnel: [w503] -> w479
      tunnel: [w502] -> w478
      tunnel: w491 -> [w515]
      tunnel: w489 -> [w514]
      tunnel: [w515] -> w495
      tunnel: [w514] -> w494
      tunnel: [w513] -> w488
      tunnel: [w512] -> w487
      tunnel: w479 -> [w507]
      tunnel: w478 -> [w506]
      tunnel: [w587] -> w493
      tunnel: w495 -> [w594]
      tunnel: w494 -> [w591]
      tunnel: w488 -> [w589]
      tunnel: w487 -> [w588]
      tunnel: [w589] -> w486
      tunnel: [w588] -> w485
      frame #0 {
        n259 = call "Loop Timer5"("Count(Ticks)"=w500) -> ("Tick Count(Ticks)"=w501:u32)
      }
      frame #1 {
        n260 = xnode "FPGA I/O Node"("Connector0/AO1"=w503, "Connector0/AO2"=w502) -> ()  [unwired: 2 in, 2 out]
      }
      frame #2 {
        n261 = local read "Scanning MCL"() -> (w527:bool)
        n262 = Or(x=w527, y="Start scan (MCL)") -> (x .or. y?=w522:bool)
        n263 = Not(x="Abort scan (MCL)") -> (.not. x?=w520:bool)
        n264 = And(x=w520, y=w522) -> (x .and. y?=w519:bool)
        n265 = case "Raster scan" shown="True" w519 {
          tunnel: [w528 w571] -> w524
          tunnel: "Start scan (MCL)" -> [_ w556]
          tunnel: [w528 w532] -> w508
          frame False {
            w528 = i16 0
            n266 = local write "Scanning MCL"(FALSE ("scanning")) -> ()
          }
          frame True {
            w542 = i16 0
            w541 = u64 0
            # "scan incr."
            # "freq. incr. mult."
            # "count steps"
            # "count number of cycles"
            n267 = feedback #28(w541) -> (w568:u64)
            n268 = Select(t=w541, s=w556, f=w568) -> (s? t:f=w570:u64)
            n269 = Increment(x=w570) -> (x+1=w567:u64)
            n270 = Greater?(x="Cycles per step (MCL)", y=w567) -> (0:w551:bool)
            n271 = Select(t=w567, s=w551, f=w541) -> (s? t:f=w566:u64)
            n272 = feedback-in #28(w566) -> ()
            n273 = feedback #29(w541) -> (w565:u64)
            n274 = Select(t=w541, s=w556, f=w565) -> (s? t:f=w560:u64)
            n275 = Increment(x=w560) -> (x+1=w564:u64)
            n276 = Add(x="Scan steps (MCL)", y="Scan steps (MCL)") -> (x+y=w563:u64)
            n277 = Select(t=w560, s=w551, f=w564) -> (s? t:f=w546:u64)
            n278 = Greater?(x=w563, y=w546) -> (0:w545:bool)
            n279 = Select(t=w546, s=w545, f=w541) -> (s? t:f=w561:u64)
            n280 = feedback-in #29(w561) -> ()
            n281 = Equal?(x="Scan steps (MCL)", y=w546) -> (x = y?=w550:bool)
            n282 = Greater?(x="Scan steps (MCL)", y=w560) -> (0:w559:bool)
            n283 = feedback #30(w542) -> (w562:i16)
            n284 = Select(t=w542, s=w556, f=w562) -> (s? t:f=w548:i16)
            n285 = Increment(x=w548) -> (x+1=w558:i16)
            n286 = Decrement(x=w548) -> (x-1=w557:i16)
            n287 = Select(t=w558, s=w559, f=w557) -> (s? t:f=w549:i16)
            n288 = Select(t=w548, s=w550, f=w549) -> (s? t:f=w547:i16)
            n289 = Select(t=w548, s=w551, f=w547) -> (s? t:f=w543:i16)
            n290 = Select(t=w543, s=w545, f=w542) -> (s? t:f=w544:i16)
            n291 = feedback-in #30(w544) -> ()
            n292 = feedback #31(w541) -> (w555:u64)
            n293 = Select(t=w541, s=w556, f=w555) -> (s? t:f=w530:u64)
            n294 = Increment(x=w530) -> (x+1=w552:u64)
            n295 = Select(t=w530, s=w545, f=w552) -> (s? t:f=w531:u64)
            n296 = Greater?(x="Number of scans (MCL)", y=w531) -> (0:w538:bool)
            n297 = Multiply(x="Scan freq.  increment (MCL)", y=w548) -> (x*y=w571:i16)
            n298 = Select(t=TRUE, s="Cont. Scan (MCL)", f=w538) -> (s? t:f=w537:bool)
            "Scanning MCL" <- w537
            n299 = Select(t=w531, s=w537, f=w541) -> (s? t:f=w553:u64)
            n300 = feedback-in #31(w553) -> ()
            n301 = Increment(x=w531) -> (x+1=→"Scan I (MCL)":u64)
            n302 = To Word Integer(number=w530) -> (16bit integer=w533:i16)
            n303 = Multiply(x=w533, y="Scan freq.  increment (MCL)") -> (x*y=w532:i16)
          }
        }
        n304 = Select(t=w508, s="1D or 2D Scan?", f=i16 0) -> (s? t:f=w509:i16)
        n305 = Select(t=w509, s="MCL Scan Axis", f=w524) -> (s? t:f=w523:i16)
        n306 = Select(t=w524, s="MCL Scan Axis", f=w509) -> (s? t:f=w525:i16)
        n307 = Add(x=w523, y="AO2") -> (x+y=w512:i16)
        n308 = Add(x="AO1", y=w525) -> (x+y=w513:i16)
        "AO1 2" <- w507
        "AO2 2" <- w506
      }
      frame #3 {
        n309 = feedback-in #32(w594) -> ()
        n310 = feedback #32(w594) -> (w593:u32)
        n311 = Boolean To (0,1)(Boolean="+ phase (MCL)") -> (0, 1=w585:i16)
        n312 = Subtract(x=w594, y=w593) -> (x-y=w592:u32)
        n313 = Multiply(x=w585, y="Phase count adjustment (MCL)") -> (x*y=w581:i16)
        n314 = Subtract(x=w592, y=w591) -> (x-y=w573:u32)
        n315 = Subtract(x="MCL count", y=w573) -> (x-y=w583:u32)
        n316 = feedback #33(i16 0) -> (w582:i16)
        n317 = Subtract(x=w582, y=w581) -> (x-y=w580:i16)
        "MCL Relative Phase" <- w580
        n318 = feedback-in #33(w580) -> ()
        n319 = Number To Boolean Array(number=w573) -> (Boolean array=w574:bool[])
        n320 = Or Array Elements(Boolean array=w574) -> (logical OR=w572:bool)
        "MCL Late?" <- w572
        n321 = Boolean To (0,1)(Boolean=w572) -> (0, 1=w579:i16)
        n322 = Add(x=w583, y=w581) -> (x+y=w587:u32)
        n323 = To Unsigned Word Integer(number=w579) -> (unsigned 16bit integer=w576:u16)
        n324 = feedback #34(u16 0) -> (w577:u16)
        n325 = Add(x=w576, y=w577) -> (x+y=w575:u16)
        "MCL Late Counter" <- w575
        n326 = feedback-in #34(w575) -> ()
      }
    }
    "Numeric" <- w480
  }
  n327 = while "RF box board direct communication loop" {
    tunnel: w2 -> [_]
    stop <- FALSE stop-if-true
    n328 = case "Whether to use direct communication method (only use one method at a time)" shown="True" "Direct RF Box \nCommunication" {
      frame False {
      }
      frame True {
        n329 = case shown="True" "Update Data" {
          frame False {
          }
          frame True {
            n330 = flat-sequence {
              frame #0 {
                n331 = First Call?() -> (First Call?: T/F=w599:bool)
                n332 = case shown="True" w599 {
                  frame False {
                  }
                  frame True {
                    # "If first time data updated, be sure to set WR high\nbefore setting data and address bits."
                    n333 = flat-sequence {
                      frame #0 {
                        n334 = xnode "FPGA I/O Node"("Connector1/DIO15"=TRUE) -> ()  [unwired: 1 in, 1 out]
                      }
                      frame #1 {
                        n335 = call "Wait"("Count(Ticks)"=u8 40 ("DO Delay 3 (Ticks)")) -> ()  [unwired: 1 out]
                      }
                    }
                  }
                }
              }
              frame #1 {
                n336 = Number To Boolean Array(number="Address") -> (Boolean array=w648:bool[])
                n337 = Number To Boolean Array(number="Data BD 1") -> (Boolean array=w649:bool[])
                n338 = Number To Boolean Array(number="Data BD 2") -> (Boolean array=w618:bool[])
                n339 = Index Array(array=w649, index=7) -> (element=w633:bool)
                n340 = Index Array(array=w649, index=6) -> (element=w632:bool)
                n341 = Index Array(array=w649, index=5) -> (element=w631:bool)
                n342 = Index Array(array=w649, index=4) -> (element=w630:bool)
                n343 = Index Array(array=w649, index=3) -> (element=w629:bool)
                n344 = Index Array(array=w649, index=2) -> (element=w628:bool)
                n345 = Index Array(array=w649, index=1) -> (element=w627:bool)
                n346 = Index Array(array=w649, index=0) -> (element=w626:bool)
                n347 = Index Array(array=w648, index=5) -> (element=w625:bool)
                n348 = Index Array(array=w648, index=4) -> (element=w624:bool)
                n349 = Index Array(array=w648, index=3) -> (element=w623:bool)
                n350 = Index Array(array=w648, index=2) -> (element=w622:bool)
                n351 = Index Array(array=w648, index=1) -> (element=w621:bool)
                n352 = Index Array(array=w648, index=0) -> (element=w620:bool)
                n353 = Index Array(array=w618, index=7) -> (element=w609:bool)
                n354 = Index Array(array=w618, index=6) -> (element=w608:bool)
                n355 = Index Array(array=w618, index=5) -> (element=w607:bool)
                n356 = Index Array(array=w618, index=4) -> (element=w606:bool)
                n357 = Index Array(array=w618, index=3) -> (element=w605:bool)
                n358 = Index Array(array=w618, index=2) -> (element=w604:bool)
                n359 = Index Array(array=w618, index=1) -> (element=w603:bool)
                n360 = Index Array(array=w618, index=0) -> (element=w602:bool)
                n361 = xnode "FPGA I/O Node"("Connector1/DIO0"=w633, "Connector1/DIO1"=w632, "Connector1/DIO2"=w631, "Connector1/DIO3"=w630, "Connector1/DIO4"=w629, "Connector1/DIO5"=w628, "Connector1/DIO6"=w627, "Connector1/DIO7"=w626, "Connector1/DIO8"=w625, "Connector1/DIO9"=w624, "Connector1/DIO10"=w623, "Connector1/DIO11"=w622, "Connector1/DIO12"=w621, "Connector1/DIO13"=w620, "Connector1/DIO20"=w609, "Connector1/DIO21"=w608, "Connector1/DIO22"=w607, "Connector1/DIO23"=w606, "Connector1/DIO24"=w605, "Connector1/DIO25"=w604, "Connector1/DIO26"=w603, "Connector1/DIO27"=w602) -> ()  [unwired: 22 in, 22 out]
              }
              frame #2 {
                # "wait and then apply write signal"
                n362 = call "Wait2"("Count(Ticks)"=u8 40 ("DO Delay 1 (Ticks)")) -> ()  [unwired: 1 out]
              }
              frame #3 {
                # "sending bit low writes data to board buffer"
                n363 = xnode "FPGA I/O Node"("Connector1/DIO15"=FALSE) -> ()  [unwired: 1 in, 1 out]
              }
              frame #4 {
                # "wait then return write signal"
                n364 = call "Wait3"("Count(Ticks)"=u8 40 ("DO Delay 2 (Ticks)")) -> ()  [unwired: 1 out]
              }
              frame #5 {
                # "sending bit high makes ready to\nwrite more data"
                n365 = xnode "FPGA I/O Node"("Connector1/DIO15"=TRUE) -> ()  [unwired: 1 in, 1 out]
              }
            }
          }
        }
      }
    }
  }
  n366 = while "Control APD data integration - stream to host" {
    shift-right: [w658] -> _
    shift-left: w2 -> [w663]
    stop <- FALSE stop-if-true
    n367 = flat-sequence {
      tunnel: w663 -> [w665]
      tunnel: [w666] -> w661
      tunnel: [w665] -> w659
      tunnel: [w674] -> w662
      tunnel: w661 -> [w674]
      tunnel: [w673] -> w660
      tunnel: w659 -> [w673]
      tunnel: [w672] -> w657
      tunnel: [w671] -> w656
      tunnel: [w708] -> w658
      tunnel: w662 -> [w720]
      tunnel: w660 -> [w717]
      tunnel: w657 -> [w701]
      tunnel: w656 -> [w700]
      frame #0 {
        n368 = call "Loop Timer6"("Count(Ticks)"=w665) -> ("Tick Count(Ticks)"=w666:u32)
      }
      frame #1 {
        n369 = flat-sequence {
          tunnel: [w676] -> w670
          tunnel: w670 -> [w678]
          tunnel: [w680] -> w669
          tunnel: [w679] -> w668
          tunnel: [w678] -> w667
          tunnel: [w686] -> w671
          tunnel: [w687] -> w672
          tunnel: w669 -> [w687]
          tunnel: w668 -> [w686]
          tunnel: w667 -> [w685]
          frame #0 {
            # "use two separate variable so each APD won't\nhave to wait to read"
            n370 = feedback #35(FALSE) -> (w675:bool)
            "APD 1 out state" <- w675
            "APD 2 out state" <- w675
            n371 = Not(x=w675) -> (.not. x?=w676:bool)
            n372 = feedback-in #35(w676) -> ()
          }
          frame #1 {
            n373 = local read "APD 1 Counts 1"() -> (w684:u32)
            n374 = local read "APD 1 Counts 0"() -> (w683:u32)
            n375 = local read "APD 2 Counts 1"() -> (w682:u32)
            n376 = local read "APD 2 Counts 0"() -> (w681:u32)
            n377 = Select(t=w684, s=w678, f=w683) -> (s? t:f=w680:u32)
            n378 = Select(t=w682, s=w678, f=w681) -> (s? t:f=w679:u32)
          }
          frame #2 {
            n379 = case shown="True" w685 {
              frame False {
                w688 = u32 0 ("APD 1 Counts 0")
                n380 = local write "APD 1 Counts 0"(w688) -> ()
                n381 = local write "APD 2 Counts 0"(w688) -> ()
              }
              frame True {
                w689 = u32 0 ("APD 1 Counts 1")
                n382 = local write "APD 1 Counts 1"(w689) -> ()
                n383 = local write "APD 2 Counts 1"(w689) -> ()
              }
            }
          }
        }
      }
      frame #2 {
        n384 = feedback-in #36(w720) -> ()
        n385 = feedback #36(w720) -> (w719:u32)
        n386 = Subtract(x=w720, y=w719) -> (x-y=w718:u32)
        n387 = Subtract(x=w718, y=w717) -> (x-y=w693:u32)
        n388 = case shown="True" "APD to FIFO" {
          tunnel: w701 -> [_ w723]
          tunnel: w700 -> [_ w721]
          frame False {
          }
          frame True {
            n389 = flat-sequence {
              tunnel: 0 ("Timeout") -> [w725]
              tunnel: w723 -> [w726]
              tunnel: [w725] -> w722
              tunnel: w722 -> [w728]
              tunnel: w721 -> [w727]
              frame #0 {
                n390 = xnode ("FIFO Write")("Element"=w726, "Timeout"=w725) -> ()  [unwired: 1 in, 2 out]
              }
              frame #1 {
                n391 = xnode ("FIFO Write")("Element"=w727, "Timeout"=w728) -> ()  [unwired: 1 in, 2 out]
              }
            }
          }
        }
        n392 = Subtract(x="APD Acq Rate Count", y=w693) -> (x-y=w709:u32)
        n393 = Number To Boolean Array(number=w693) -> (Boolean array=w694:bool[])
        n394 = Or Array Elements(Boolean array=w694) -> (logical OR=w692:bool)
        "APD Acq Late?" <- w692
        n395 = Boolean To (0,1)(Boolean=w692) -> (0, 1=w699:i16)
        n396 = To Unsigned Word Integer(number=w699) -> (unsigned 16bit integer=w696:u16)
        n397 = Boolean To (0,1)(Boolean="+ phase (APD Acq)") -> (0, 1=w705:i16)
        n398 = feedback #37(u16 0) -> (w697:u16)
        n399 = Add(x=w696, y=w697) -> (x+y=w695:u16)
        "APD Acq Late Counter" <- w695
        n400 = feedback-in #37(w695) -> ()
        n401 = Multiply(x=w705, y="Phase Count Adjustment (APD Acq)") -> (x*y=w702:i16)
        n402 = Add(x=w709, y=w702) -> (x+y=w708:u32)
        n403 = feedback #38(i16 0) -> (w707:i16)
        n404 = Subtract(x=w707, y=w702) -> (x-y=w704:i16)
        "APD Acq Relative Phase" <- w704
        n405 = feedback-in #38(w704) -> ()
        n406 = To Word Integer(number=w701) -> (16bit integer=w710:i16)
        n407 = To Word Integer(number=w700) -> (16bit integer=w711:i16)
        n408 = Multiply(x="APD 1 AO scale factor", y=w710) -> (x*y=w691:i16)
        n409 = Multiply(x="APD 2 AO scale factor", y=w711) -> (x*y=w690:i16)
        n410 = xnode "FPGA I/O Node"("Connector0/AO5"=w691, "Connector0/AO7"=w690) -> ()  [unwired: 2 in, 2 out]
      }
    }
  }
  n411 = while "RF box board DIO control: parallel communication" {
    shift-right: [w735] -> _
    shift-left: w2 -> [w734]
    shift-right: [w733] -> _
    shift-left: FALSE ("Swap F1 and F2") -> [w732]
    stop <- FALSE stop-if-true
    n412 = flat-sequence {
      tunnel: w732 -> [w739]
      tunnel: w734 -> [w737]
      tunnel: [w739] -> w731
      tunnel: [w738] -> w730
      tunnel: [w737] -> w729
      tunnel: [w745] -> w735
      tunnel: [w744] -> w733
      tunnel: w731 -> [w743]
      tunnel: w730 -> [w741]
      tunnel: w729 -> [w740]
      frame #0 {
        n413 = call "Loop Timer"("Count(Ticks)"=w737) -> ("Tick Count(Ticks)"=w738:u32)
      }
      frame #1 {
        n414 = flat-sequence {
          tunnel: ["FPGA Controls\n RF Box"] -> w742
          tunnel: w743 -> [w746]
          tunnel: [w786] -> w745
          tunnel: [w799] -> w744
          tunnel: w742 -> [w798]
          tunnel: w741 -> [w792]
          tunnel: w740 -> [w789]
          frame #0 {
            n415 = case shown="True" "FPGA Controls\n RF Box" {
              tunnel: w746 -> [_ w748]
              frame False {
              }
              frame True {
                n416 = flat-sequence {
                  tunnel: w748 -> [w754]
                  frame #0 {
                    n417 = First Call?() -> (First Call?: T/F=w749:bool)
                    n418 = case shown="True" w749 {
                      frame False {
                      }
                      frame True {
                        # "If first time data updated, be sure to set WR high and UDCLK low\nbefore setting data and address bits."
                        n419 = xnode "FPGA I/O Method Node"("Enable"=TRUE) -> ("FPGA I/O Out"=w751:refnum<k21>)  [unwired: 1 in]
                        n420 = xnode "FPGA I/O Node"("Connector1/DIO15"=TRUE) -> ()  [unwired: 1 in, 1 out]
                        n421 = xnode "FPGA I/O Node"("I/O Item"=FALSE ("Connector1/DIO30"), "FPGA I/O In"=w751) -> ()  [unwired: 1 out]
                      }
                    }
                  }
                  frame #1 {
                    n422 = case shown="True" "Freq or Amp switch first" {
                      tunnel: w754 -> [w756 w761]
                      frame False {
                        n423 = flat-sequence {
                          tunnel: w756 -> [w760]
                          frame #0 {
                            # "switch amplitude"
                            # "send udclk high"
                            n424 = xnode "FPGA I/O Node"("Connector1/DIO30"=TRUE ("Connector1/DIO15")) -> ()  [unwired: 1 in, 1 out]
                          }
                          frame #1 {
                            # "send udclk low"
                            n425 = xnode "FPGA I/O Node"("Connector1/DIO30"=FALSE ("Connector1/DIO15")) -> ()  [unwired: 1 in, 1 out]
                          }
                          frame #2 {
                            n426 = call "Wait5"("Count(Ticks)"="Freq switch delay") -> ()  [unwired: 1 out]
                          }
                          frame #3 {
                            # "switch frequency"
                            n427 = xnode "FPGA I/O Node"("Connector1/DIO36"=w760) -> ()  [unwired: 1 in, 1 out]
                          }
                        }
                      }
                      frame True {
                        n428 = flat-sequence {
                          tunnel: w761 -> [w762]
                          frame #0 {
                            # "switch frequency"
                            n429 = xnode "FPGA I/O Node"("Connector1/DIO36"=w762) -> ()  [unwired: 1 in, 1 out]
                          }
                          frame #1 {
                            n430 = call "Wait4"("Count(Ticks)"="Amp switch delay") -> ()  [unwired: 1 out]
                          }
                          frame #2 {
                            # "switch amplitude"
                            # "send udclk high"
                            n431 = xnode "FPGA I/O Node"("Connector1/DIO30"=TRUE ("Connector1/DIO15")) -> ()  [unwired: 1 in, 1 out]
                          }
                          frame #3 {
                            # "send udclk low"
                            n432 = xnode "FPGA I/O Node"("Connector1/DIO30"=FALSE ("Connector1/DIO15")) -> ()  [unwired: 1 in, 1 out]
                          }
                        }
                      }
                    }
                  }
                }
              }
            }
          }
          frame #1 {
            # "This is the prior cycle's on time"
            # "increment timing\nindex, reset to 0 if \nend of matrix"
            # "Reset to begginning (1) when number of cycles reached."
            # "timing index"
            # "build byte stacks for writing data\n(must correspond to addresses array constant)"
            # "Timing housekeeping"
            # "Adjust phase if late\n(maintains constant phase relationship between cycles)"
            n433 = feedback #39(u8 0 ("t")) -> (w795:u8)
            n434 = Increment(x=w795) -> (x+1=w839:u8)
            n435 = Increment(x="Number Interlace Cycles") -> (x+1=w834:u8)
            n436 = Equal?(x=w839, y=w834) -> (x = y?=w841:bool)
            n437 = Select(t=u8 1, s=w841, f=w839) -> (s? t:f=w794:u8)
            n438 = feedback-in #39(w794) -> ()
            n439 = Increment(x=w794) -> (x+1=w836:u8)
            n440 = Equal?(x=w836, y=w834) -> (x = y?=w837:bool)
            n441 = Select(t=u8 1, s=w837, f=w836) -> (s? t:f=w833:u8)
            n442 = Select(t=w833, s="Interlace ON/OFF", f="Interlace Off Parameters") -> (s? t:f=w817:u8)
            n443 = case shown="1, Default" w817 {
              tunnel: [w911 w1076 "BD 1 Frequency 3"] -> w829
              tunnel: [w910 "BD 2 Frequency 2" "BD 2 Frequency 3"] -> w818
              tunnel: ["BD 2 Amplitude 1" "BD 2 Amplitude 2" "BD 2 Amplitude 3"] -> w774
              tunnel: [w900 w1086 "BD 1 Amplitude 3"] -> w777
              frame 1, Default {
                w891 = fxp<+/-,24,9> 0.0 ("AI1 X Set 2")
                w884 = u16 0
                w906 = u64 0 ("f")
                # "This signal integration happens no matter what\nso that correct setpoints can be chosen before \nturning on the FB."
                # "Trap 1"
                n444 = local read "AI1 X Set 2"() -> (w887:fxp<+/-,16,1>)
                n445 = local read "AI1 X Set 1"() -> (w888:fxp<+/-,16,1>)
                n446 = local read "Scanning"() -> (w912:bool)
                n447 = case shown="False" "Diff FB Measurement?" {
                  tunnel: w887 -> [w920 w929]
                  tunnel: w888 -> [w919 w930]
                  tunnel: [w917 w921] -> w889
                  frame False {
                    n448 = Select(t=w919, s="Trap Pos FB Monitor T1 or T2", f=w920) -> (s? t:f=w917:fxp<+/-,16,1>)
                  }
                  frame True {
                    n449 = Subtract(x=w930, y=w929) -> (x-y=w922:fxp<+/-,17,2>)
                    n450 = Not(x="Negate Diff?") -> (.not. x?=w928:bool)
                    n451 = Boolean To (0,1)(Boolean="Negate Diff?") -> (0, 1=w926:i16)
                    n452 = Boolean To (0,1)(Boolean=w928) -> (0, 1=w927:i16)
                    n453 = Negate(x=w926) -> (-x=w925:i16)
                    n454 = Add(x=w925, y=w927) -> (x+y=w923:i16)
                    n455 = Multiply(x=w923, y=w922) -> (x*y=w921:fxp<+/-,32,17>)
                  }
                }
                n456 = Or(x=w912, y="Start scan") -> (x .or. y?=w904:bool)
                n457 = Not(x="Abort scan") -> (.not. x?=w902:bool)
                n458 = And(x=w902, y=w904) -> (x .and. y?=w875:bool)
                n459 = feedback #40(w884) -> (w883:u16)
                n460 = Increment(x=w883) -> (x+1=w885:u16)
                n461 = Greater Or Equal?(x=w885, y="Trap Pos FB Int Count") -> (x >= y?=w876:bool)
                n462 = case "For raster scanning" shown="False" w875 {
                  tunnel: [w1017 w1029] -> w907
                  tunnel: "Start scan" -> [_ w1053]
                  frame False {
                    # "For wiggle-calibration: sinusoidal wave"
                    n463 = local read "Wiggling 1"() -> (w1012:bool)
                    n464 = Not(x="Abort wiggle 1") -> (.not. x?=w1015:bool)
                    n465 = Or(x="Wiggle trap 1", y=w1012) -> (x .or. y?=w1011:bool)
                    n466 = And(x=w1011, y=w1015) -> (x .and. y?=w1014:bool)
                    n467 = case shown="True" w1014 {
                      tunnel: [u64 0 w1025] -> w1017
                      frame False {
                        n468 = local write "Wiggling 1"(FALSE ("Wiggle")) -> ()
                      }
                      frame True {
                        # "Input is periods/tick, not Hz,\nso need to normalize by clock\nfrequency (40 MHz)."
                        n469 = Divide(x="Wiggle freq 1 (Hz)", y=fxp<+,17,26> 40000000.0) -> (x/y=w1022:fxp<+/-,17,-9>)
                        n470 = call "Sine Wave Generator"("frequency (periods/tick)"=w1022) -> ("sine out"=w1027:i32)  [unwired: 14 in]
                        n471 = Multiply(x=w1027, y="Wiggle amp 1") -> (x*y=w1025:u64)
                        "Wiggling 1" <- TRUE
                      }
                    }
                    n472 = local write "Scanning"(FALSE ("scanning")) -> ()
                  }
                  frame True {
                    w1037 = i64 0
                    w1036 = u64 0
                    # "scan incr."
                    # "freq. incr. mult."
                    # "count steps"
                    # "count number of cycles"
                    n473 = feedback #41(w1036) -> (w1065:u64)
                    n474 = Select(t=w1036, s=w1053, f=w1065) -> (s? t:f=w1067:u64)
                    n475 = Increment(x=w1067) -> (x+1=w1064:u64)
                    n476 = Greater?(x="Cycles per step", y=w1064) -> (0:w1046:bool)
                    n477 = Select(t=w1064, s=w1046, f=w1036) -> (s? t:f=w1063:u64)
                    n478 = feedback-in #41(w1063) -> ()
                    n479 = feedback #42(w1036) -> (w1062:u64)
                    n480 = Select(t=w1036, s=w1053, f=w1062) -> (s? t:f=w1057:u64)
                    n481 = Increment(x=w1057) -> (x+1=w1061:u64)
                    n482 = Add(x="Scan steps", y="Scan steps") -> (x+y=w1060:u64)
                    n483 = Select(t=w1057, s=w1046, f=w1061) -> (s? t:f=w1041:u64)
                    n484 = Greater?(x=w1060, y=w1041) -> (0:w1040:bool)
                    n485 = Select(t=w1041, s=w1040, f=w1036) -> (s? t:f=w1058:u64)
                    n486 = feedback-in #42(w1058) -> ()
                    n487 = Equal?(x="Scan steps", y=w1041) -> (x = y?=w1045:bool)
                    n488 = Greater?(x="Scan steps", y=w1057) -> (0:w1056:bool)
                    n489 = feedback #43(w1037) -> (w1059:i64)
                    n490 = Select(t=w1037, s=w1053, f=w1059) -> (s? t:f=w1043:i64)
                    n491 = Increment(x=w1043) -> (x+1=w1055:i64)
                    n492 = Decrement(x=w1043) -> (x-1=w1054:i64)
                    n493 = Select(t=w1055, s=w1056, f=w1054) -> (s? t:f=w1044:i64)
                    n494 = Select(t=w1043, s=w1045, f=w1044) -> (s? t:f=w1042:i64)
                    n495 = Select(t=w1043, s=w1046, f=w1042) -> (s? t:f=w1038:i64)
                    n496 = Select(t=w1038, s=w1040, f=w1037) -> (s? t:f=w1039:i64)
                    n497 = feedback-in #43(w1039) -> ()
                    n498 = feedback #44(w1036) -> (w1052:u64)
                    n499 = Select(t=w1036, s=w1053, f=w1052) -> (s? t:f=w1048:u64)
                    n500 = Increment(x=w1048) -> (x+1=w1049:u64)
                    n501 = Select(t=w1048, s=w1040, f=w1049) -> (s? t:f=w1047:u64)
                    n502 = Greater?(x="Number of scans", y=w1047) -> (0:w1033:bool)
                    n503 = Multiply(x="Scan freq.  increment", y=w1043) -> (x*y=w1029:i64)
                    n504 = Select(t=TRUE, s="Cont. Scan", f=w1033) -> (s? t:f=w1032:bool)
                    "Scanning" <- w1032
                    n505 = Select(t=w1047, s=w1032, f=w1036) -> (s? t:f=w1050:u64)
                    n506 = feedback-in #44(w1050) -> ()
                    n507 = Increment(x=w1047) -> (x+1=→"Scan I":u64)
                  }
                }
                n508 = Select(t=w884, s=w876, f=w885) -> (s? t:f=w886:u16)
                n509 = feedback-in #40(w886) -> ()
                n510 = feedback #45(w891) -> (w890:fxp<+/-,24,9>)
                n511 = Add(x=w889, y=w890) -> (x+y=w882:fxp<+/-,24,9>)
                n512 = Select(t=w891, s=w876, f=w882) -> (s? t:f=w894:fxp<+/-,24,9>)
                n513 = feedback-in #45(w894) -> ()
                n514 = Divide(x=w882, y="Trap Pos FB Int Count") -> (x/y=w877:fxp<+/-,16,1>)
                n515 = feedback #46(fxp<+/-,24,9> 0.0 ("AI1 X Set 2")) -> (w895:fxp<+/-,24,9>)
                n516 = Select(t=w882, s=w876, f=w895) -> (s? t:f=w896:fxp<+/-,24,9>)
                "Trap Pos FB Int Signal" <- w896
                n517 = feedback-in #46(w896) -> ()
                n518 = feedback #47(fxp<+/-,16,1> 0.0 ("Trap Pos FB Int-Norm Signal")) -> (w879:fxp<+/-,16,1>)
                n519 = Select(t=w877, s=w876, f=w879) -> (s? t:f=w878:fxp<+/-,16,1>)
                "Trap Pos FB Int-Norm Signal" <- w878
                n520 = feedback-in #47(w878) -> ()
                n521 = case "For position feedback" shown="True" "Force feedback" {
                  tunnel: [i64 0 w936] -> w897
                  tunnel: w877 -> [_ w933]
                  tunnel: w876 -> [_ w932]
                  frame False {
                  }
                  frame True {
                    n522 = feedback #48(i64 0) -> (w935:i64)
                    n523 = case shown="True" w932 {
                      tunnel: [w937 w944] -> w936
                      tunnel: w935 -> [w937 _]
                      tunnel: w933 -> [_ w938]
                      frame False {
                      }
                      frame True {
                        w948 = u32 0
                        n524 = xnode ("PID")("process variable"=w938, "reset?"="Trap Pos. FB Reset", "setpoint"="Trap Pos. FB SP", "PID gains"="Trap Pos. FB Gains", "output range"="Trap Pos. FB Range") -> ("output"=w960:fxp<+/-,16,1>)
                        n525 = Negate(x=w960) -> (-x=w959:fxp<+/-,17,2>)
                        n526 = Select(t=w959, s="Trap Pos FB Negate Action", f=w960) -> (s? t:f=w956:fxp<+/-,17,2>)
                        n527 = Scale By Power Of 2(n=u32 15, x=u32 1) -> (x*2^n=w953:u32)
                        n528 = Multiply(x=w956, y=w953) -> (x*y=w952:fxp<+/-,17,17>)
                        n529 = To Quad Integer(1:w952) -> (0:w964:i64)
                        "Trap Pos FB Action" <- w964
                        n530 = Multiply(x=w964, y="Trap Pos. FB Mult Factor") -> (x*y=w962:i64)
                        n531 = Add(x=w962, y="Trap Pos. FB Offset Factor") -> (x+y=w944:i64)
                        n532 = feedback #49() -> (w945:i64)  [unwired: 1 in]
                        n533 = Add(x=w944, y=w945) -> (x+y=w942:i64)
                        n534 = feedback #50(w948) -> (w950:u32)
                        n535 = Increment(x=w950) -> (x+1=w939:u32)
                        n536 = Greater Or Equal?(x=w939, y="FB Trig Integrate") -> (x >= y?=w940:bool)
                        n537 = Select(t=i64 0, s=w940, f=w942) -> (s? t:f=w946:i64)
                        n538 = feedback-in #49(w946) -> ()
                        n539 = Select(t=w948, s=w940, f=w939) -> (s? t:f=w949:u32)
                        n540 = feedback-in #50(w949) -> ()
                        n541 = And(x=w940, y="FPGA Trap Trig") -> (x .and. y?=w947:bool)
                        n542 = case "Trap FB trigger excitation laser ON" shown="True" w947 {
                          tunnel: w942 -> [_ w970]
                          tunnel: w939 -> [_ w968]
                          frame False {
                          }
                          frame True {
                            n543 = Not(x="TTrig Negate Pos") -> (.not. x?=w977:bool)
                            n544 = Boolean To (0,1)(Boolean="TTrig Negate Pos") -> (0, 1=w975:i16)
                            n545 = Boolean To (0,1)(Boolean=w977) -> (0, 1=w976:i16)
                            n546 = Negate(x=w975) -> (-x=w974:i16)
                            n547 = Add(x=w974, y=w976) -> (x+y=w973:i16)
                            n548 = Multiply(x=w973, y=w970) -> (x*y=w972:i64)
                            "TTrig Sig" <- w972
                            n549 = Multiply(x="FPGA TTrig Thresh", y=w968) -> (x*y=w969:i64)
                            "TTrig Fin Thresh" <- w969
                            n550 = Greater Or Equal?(x=w972, y=w969) -> (x >= y?=w971:bool)
                            n551 = case shown="True" w971 {
                              frame False {
                              }
                              frame True {
                                w980 = TRUE ("Green FB On/Off")
                                w982 = u8 2 ("Operating Mode")
                                n552 = local write "Operating Mode 2"(w982) -> ()
                                n553 = local write "Operating Mode"(w982) -> ()
                                n554 = local write "Green FB On/Off"(w980) -> ()
                                n555 = local write "FPGA Trap Trig"(FALSE ("FPGA Trap Trig")) -> ()
                                "TTrig?" <- w980
                              }
                            }
                          }
                        }
                      }
                    }
                    n556 = feedback-in #48(w936) -> ()
                  }
                }
                n557 = case "For intensity feedback" shown="True" "FB On/Off Set 1" {
                  tunnel: "BD 1 Amplitude 1" -> [w1068 _]
                  tunnel: [w1068 w1069] -> w900
                  frame False {
                  }
                  frame True {
                    n558 = local read "AI2 Y Sum Set 1"() -> (w1071:i16)
                    n559 = call "Slower PID.vi"("process variable"=w1071, "reset?"="FB Reset Set 1", "setpoint"="FB Setpoint Set 1", "PID gains (x 2^8)"="FB Gains Set 1", "output range"="FB output range 1") -> ("output"=w1074:i16)  [unwired: 10 out]
                    n560 = To Unsigned Word Integer(number=w1074) -> (unsigned 16bit integer=w1069:u16)
                  }
                }
                n561 = Select(t=w906, s="Scan BD", f=w907) -> (s? t:f=w905:u64)
                n562 = Select(t=w907, s="Scan BD", f=w906) -> (s? t:f=w908:u64)
                n563 = Add(x=w905, y="BD 2 Frequency 1") -> (x+y=w910:u64)
                n564 = Compound Arithmetic op=ADD("BD 1 Frequency 1", w897, w908) -> (w911:u64)
                "BD1 Frequency Out 1" <- w911
              }
              frame 2 {
                # "For wiggle calibration"
                # "Trap 2"
                n565 = local read "Wiggling 2"() -> (w1083:bool)
                n566 = Or(x="Wiggle trap 2", y=w1083) -> (x .or. y?=w1082:bool)
                n567 = Not(x="Abort wiggle 2") -> (.not. x?=w1080:bool)
                n568 = And(x=w1082, y=w1080) -> (x .and. y?=w1079:bool)
                n569 = case shown="True" "FB On/Off Set 2" {
                  tunnel: [w1099 w1100] -> w1086
                  tunnel: "BD 1 Amplitude 2" -> [w1099 _]
                  frame False {
                  }
                  frame True {
                    n570 = local read "AI2 Y Sum Set 2"() -> (w1105:i16)
                    n571 = call "Slower PID.vi"("process variable"=w1105, "reset?"="FB Reset Set 2", "setpoint"="FB Setpoint Set 2", "PID gains (x 2^8)"="FB Gains Set 2", "output range"="FB output range 2") -> ("output"=w1102:i16)  [unwired: 10 out]
                    n572 = To Unsigned Word Integer(number=w1102) -> (unsigned 16bit integer=w1100:u16)
                  }
                }
                n573 = case shown="True" w1079 {
                  tunnel: [i16 0 w1093] -> w1077
                  frame False {
                    n574 = local write "Wiggling 2"(FALSE) -> ()
                  }
                  frame True {
                    n575 = Divide(x="Wiggle freq 2 (Hz)", y=fxp<+,17,26> 40000000.0) -> (x/y=w1096:fxp<+/-,17,-9>)
                    n576 = call "Sine Wave Generator2"("frequency (periods/tick)"=w1096) -> ("sine out"=w1095:i32)  [unwired: 14 in]
                    n577 = Multiply(x=w1095, y="Wiggle amp 2") -> (x*y=w1093:u64)
                    "Wiggling 2" <- TRUE
                  }
                }
                n578 = Add(x="BD 1 Frequency 2", y=w1077) -> (x+y=w1076:u64)
                "BD1 Frequency Out 2" <- w1076
              }
              frame 3 {
                # "Fluorescence period"
              }
            }
            n579 = feedback-in #51(w792) -> ()
            n580 = feedback #51(w792) -> (w791:u32)
            n581 = Select(t=w794, s="Interlace ON/OFF", f="Interlace Off Parameters") -> (s? t:f=w832:u8)
            n582 = Subtract(x=w792, y=w791) -> (x-y=w790:u32)
            n583 = Subtract "The error"(x=w790, y=w789) -> (x-y=w767:u32)
            n584 = case shown="1, Default" w832 {
              tunnel: ["DIO count 1 (ticks)" "DIO count 2 (ticks)" "DIO count 3 (ticks)"] -> w788
              frame 1, Default {
              }
              frame 2 {
              }
              frame 3 {
              }
            }
            n585 = Number To Boolean Array(number=w767) -> (Boolean array=w768:bool[])
            n586 = Or Array Elements(Boolean array=w768) -> (logical OR=w766:bool)
            "DIO Late?" <- w766
            n587 = Boolean To (0,1)(Boolean=w766) -> (0, 1=w773:i16)
            n588 = To Unsigned Word Integer(number=w773) -> (unsigned 16bit integer=w770:u16)
            n589 = feedback #52(u16 0) -> (w771:u16)
            n590 = Add(x=w770, y=w771) -> (x+y=w769:u16)
            "DIO Late Counter" <- w769
            n591 = feedback-in #52(w769) -> ()
            n592 = Subtract(x=w788, y=w767) -> (x-y=w787:u32)
            n593 = Split Number(x=w829) -> (hi(x)=w828:u32, lo(x)=w827:u32)
            n594 = Split Number(x=w818) -> (hi(x)=w823:u32, lo(x)=w822:u32)
            n595 = Boolean To (0,1)(Boolean="+ phase (DIO)") -> (0, 1=w784:i16)
            n596 = Split Number(x=w828) -> (lo(x)=w826:u16)  [unwired: 1 out]
            n597 = Split Number(x=w827) -> (hi(x)=w825:u16, lo(x)=w824:u16)
            n598 = Split Number(x=w823) -> (lo(x)=w821:u16)  [unwired: 1 out]
            n599 = Split Number(x=w822) -> (hi(x)=w820:u16, lo(x)=w819:u16)
            n600 = Split Number(x=w777) -> (hi(x)=w779:u8, lo(x)=w778:u8)
            n601 = Split Number(x=w774) -> (hi(x)=w776:u8, lo(x)=w775:u8)
            n602 = Split Number(x=w826) -> (hi(x)=w816:u8, lo(x)=w815:u8)
            n603 = Split Number(x=w825) -> (hi(x)=w814:u8, lo(x)=w813:u8)
            n604 = Split Number(x=w821) -> (hi(x)=w809:u8, lo(x)=w808:u8)
            n605 = Split Number(x=w824) -> (hi(x)=w812:u8, lo(x)=w811:u8)
            n606 = Split Number(x=w820) -> (hi(x)=w807:u8, lo(x)=w806:u8)
            n607 = Split Number(x=w819) -> (hi(x)=w805:u8, lo(x)=w804:u8)
            n608 = Multiply(x=w784, y="Phase count adjustment (DIO)") -> (x*y=w780:i16)
            n609 = feedback #53(i16 0) -> (w782:i16)
            n610 = Subtract(x=w782, y=w780) -> (x-y=w781:i16)
            "DIO Relative phase" <- w781
            n611 = feedback-in #53(w781) -> ()
            n612 = Add(x=w787, y=w780) -> (x+y=w786:u32)
            n613 = Build Array "BD 1 A Stack"(w779, w778) -> (w801:u8[])
            n614 = Build Array "BD 2 A Stack"(w776, w775) -> (w800:u8[])
            n615 = Build Array "BD 1 nu Stack"(w816, w815, w814, w813, w812, w811) -> (w810:u8[])
            n616 = Build Array "BD 2 nu Stack"(w809, w808, w807, w806, w805, w804) -> (w803:u8[])
            n617 = case shown="2" w817 {
              tunnel: [w867 w870] -> w799
              tunnel: [u8 10 u8 4] -> w802
              tunnel: "Swap F1 and F2" -> [w868 w870]
              frame 2 {
                # "F2"
                n618 = Not(x=w868) -> (.not. x?=w867:bool)
              }
              frame 1, Default {
                # "low chooses F1"
                # "F1"
              }
            }
            n619 = case "If FPGA is controlling (toggling) RF synth" shown="True" w798 {
              tunnel: w810 -> [_ w846]
              tunnel: w803 -> [_ w845]
              tunnel: w802 -> [_ w844]
              tunnel: w801 -> [_ w843]
              tunnel: w800 -> [_ w842]
              frame False {
              }
              frame True {
                # "Write next amp.\n(wait until beginning of next loop iteration to update)"
                n620 = flat-sequence "Update the next F1 and F2 frequency value (the actual frequency won't change until FSK is switched).\nThen load the next amplitude value into buffer, but don't update it until the next cycle." {
                  tunnel: w846 -> [w849]
                  tunnel: w845 -> [w848]
                  tunnel: w844 -> [w847]
                  tunnel: w843 -> [w860]
                  tunnel: w842 -> [w859]
                  frame #0 {
                    n621 = for {
                      tunnel: w849 -> [w855] mode=indexing
                      tunnel: w848 -> [w854] mode=indexing
                      tunnel: w847 -> [w852]
                      i -> [w853]
                      # "Write next freq."
                      n622 = To Unsigned Byte Integer(number=w853) -> (unsigned 8bit integer=w850:u8)
                      n623 = Add(x=w852, y=w850) -> (x+y=w851:u8)
                      n624 = call "write to RF synth bd.vi"("Address Byte"=w851, "BD 2 Byte"=w854, "BD 1 Byte"=w855) -> ()
                    }
                  }
                  frame #1 {
                    # "send udclk high"
                    n625 = xnode "FPGA I/O Node"("Connector1/DIO30"=TRUE ("Connector1/DIO15")) -> ()  [unwired: 1 in, 1 out]
                  }
                  frame #2 {
                    n626 = xnode "FPGA I/O Node"("Connector1/DIO30"=FALSE ("Connector1/DIO15")) -> ()  [unwired: 1 in, 1 out]
                  }
                  frame #3 {
                    n627 = for {
                      tunnel: w860 -> [w866] mode=indexing
                      tunnel: w859 -> [w865] mode=indexing
                      tunnel: u8 33 -> [w863]
                      i -> [w864]
                      n628 = To Unsigned Byte Integer(number=w864) -> (unsigned 8bit integer=w861:u8)
                      n629 = Add(x=w863, y=w861) -> (x+y=w862:u8)
                      n630 = call "write to RF synth bd.vi"("Address Byte"=w862, "BD 2 Byte"=w865, "BD 1 Byte"=w866) -> ()
                    }
                  }
                }
              }
            }
          }
        }
      }
    }
  }
  n631 = node-c288(w4) -> ()
